vi "Discover Network Analyzer Model.vi"(10 "Model In":string) -> (2 "selection":bool)   [LabVIEW 2018]
panel:
  out "size(s)":i32
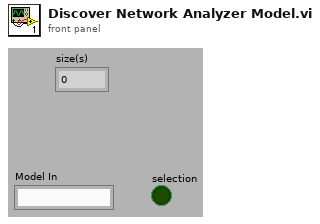
[diagram p1: front panel]
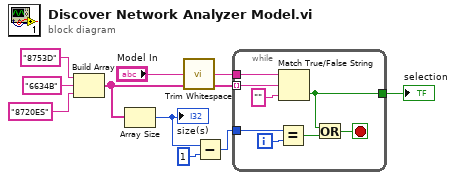
[diagram p0: block diagram]
diagram:
  n1 = Build Array("8753D" ("true string"), "6634B" ("true string"), "8720ES" ("element")) -> (w7:string[])
  n2 = Array Size(array=w7) -> (size(s)=w6:i32)
  "size(s)" <- w6
  n3 = call <vilib>:"Trim Whitespace.vi"("string"="Model In") -> ("trimmed string"=w2:string)  [unwired: 1 in]
  n4 = Subtract(x=w6, y=1) -> (x-y=w4:i32)
  n5 = while {
    tunnel: w7 -> [w17] mode=indexing
    tunnel: w2 -> [w16]
    tunnel: [w15] -> w8
    tunnel: w4 -> [w11]
    i -> [w12]
    stop <- w14 stop-if-true
    n6 = Equal?(x=w11, y=w12) -> (x = y?=w13:bool)
    n7 = Match True/False String(2:"" ("false string"), 3:w17, 4:w16) -> (0:w15:bool)  [unwired: 1 out]
    n8 = Or(x=w15, y=w13) -> (x .or. y?=w14:bool)
  }
  "selection" <- w8
